vi "Vision Assistant.vi"(0 "Color Plane (Color Plane Extraction 1)":i32(ring)=2 items=["Red", "Green", "Blue", "Hue", "Saturation", "Luminance", "Value", "Intensity"], 1 "Range (Threshold 1)":cluster{"Lower value":sgl, "Upper value":sgl}={"Lower value"=199.0, "Upper value"=255.0}, 2 "Number of Erosion (Adv. Morphology 1)":i32=1, 3 "Square/Hexa (Square) (Adv. Morphology 1)":bool, 4 "Connectivity 4/8 (8) (Adv. Morphology 1)":bool=TRUE, 5 "Low Pass/High Pass (Low) (Adv. Morphology 1)":bool, 7 "error in":errorcluster) -> (20 "Number of Matches (Shape Matching 1)":i32, 21 "Shape Report (calibrated) (Shape Matching 1)":T2(array[cluster]) {"Score" format="%.2f"; "Centroid"."y" format="%.2f"; "Centroid"."x" format="%.2f"}, 27 "error out":errorcluster)   [LabVIEW 2016]
uses:
  <vilib>/vision/NI_Vision_Development_Module.lvlib
panel:
  out "Image Out":T1(plugin-control)
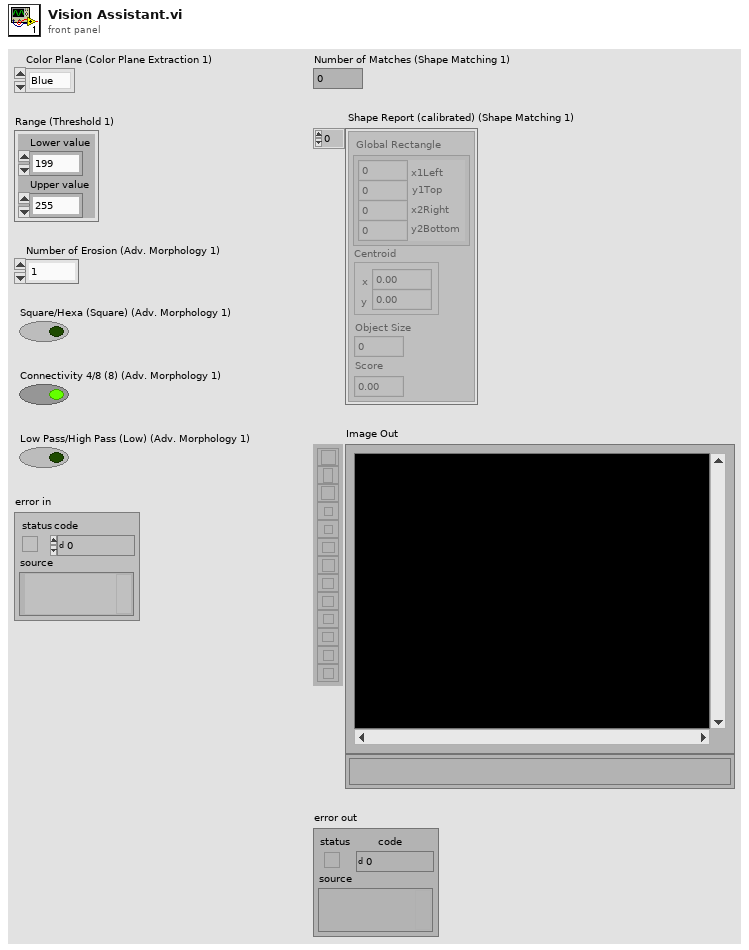
[diagram p1: front panel]
types:
  T1 = typedef "IMAQ Image.ctl" = refnum<image>
  T2 = cluster{"Global Rectangle":cluster{"x1Left":i32, "y1Top":i32, "x2Right":i32, "y2Bottom":i32}, "Centroid":cluster{"x":sgl, "y":sgl}, "Object Size":u32, "Score":dbl}[]
  T3 = typedef "Image Type" = u32
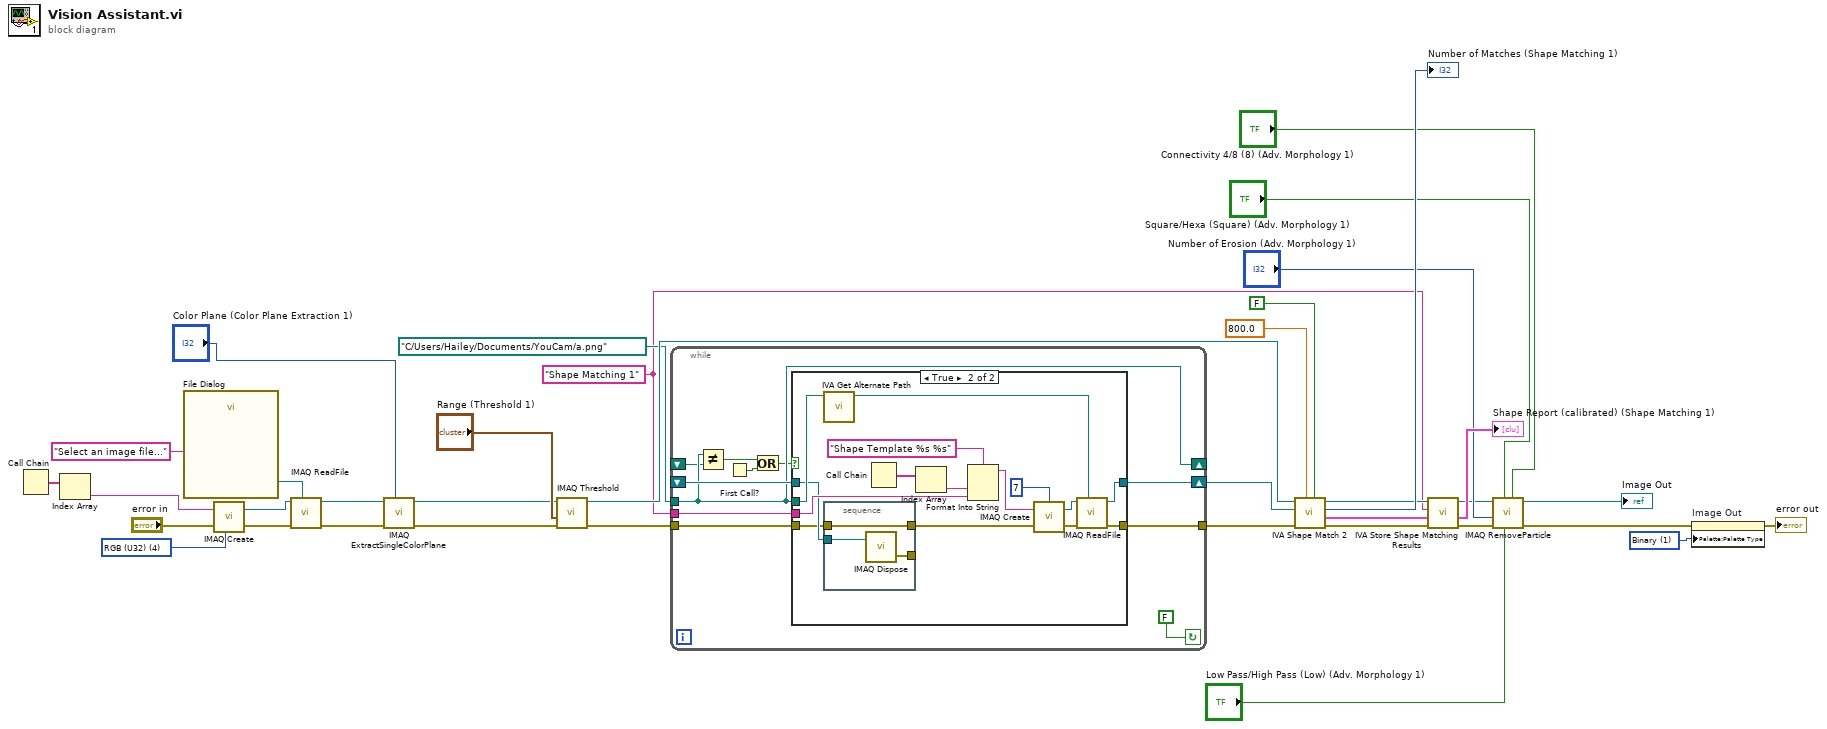
[diagram p0: block diagram]
diagram:
  w1 = u32 1 items=["Grayscale", "Binary", "Gradient", "Rainbow", "Temperature", "User Defined", "Binary 16 Bit", "Gradient 16 Bit", "Rainbow 16 Bit", "Temperature 16 Bit", "User Defined 16 Bit"] ("Palette Type")
  w10 = "Shape Matching 1" ("Step Name")
  w29 = T3 4 items=["Grayscale (U8)", "Grayscale (I16)", "Grayscale (SGL)", "Complex (CSG)", "RGB (U32)", "HSL (U32)", "RGB (U64)", "Grayscale (U16)"] ("Image Type")
  n1 = Call Chain() -> (call chain=w33:string[])
  n2 = Index Array(array=w33) -> (element=w32:string)  [unwired: 1 in]
  n3 = call "File Dialog"("prompt"="Select an image file...") -> ("selected path"=w30:path)  [unwired: 6 in, 8 out]
  n4 = call "IMAQ Create"("Image Name"=w32, "Image Type"=w29, "error in (no error)"="error in") -> ("New Image"=w36:T1, "error out"=w35:errorcluster)  [unwired: 1 in, 1 out]
  n5 = call "IMAQ ReadFile"("File Path"=w30, "error in (no error)"=w35, "Image"=w36) -> ("error out"=w37:errorcluster, "Image Out"=w27:T1)  [unwired: 2 in, 5 out]
  n6 = call "IMAQ ExtractSingleColorPlane"("Color Plane"="Color Plane (Color Plane Extraction 1)", "error in (no error)"=w37, "Image Src"=w27) -> ("error out"=w26:errorcluster, "Image Dst Out"=w24:T1)  [unwired: 1 in, 6 out]
  n7 = call "IMAQ Threshold"("error in (no error)"=w26, "Range"="Range (Threshold 1)", "Image Src"=w24) -> ("error out"=w23:errorcluster, "Image Dst Out"=w19:T1)  [unwired: 3 in, 4 out]
  n8 = while {
    shift-right: [w48] -> w11
    shift-left: _ -> [w47]
    tunnel: [w45] -> w12
    tunnel: w23 -> [w44]
    tunnel: path "C:/Users/Hailey/Documents/YouCam/a.png" ("Template Path") -> [w42]
    tunnel: w10 -> [w43]
    shift-right: [w42] -> _
    shift-left: _ -> [w41]
    stop <- FALSE continue-if-true
    n9 = Not Equal?(x=w42, y=w41) -> (x != y?=w39:bool)
    n10 = First Call?() -> (First Call?: T/F=w40:bool)
    n11 = Or(x=w39, y=w40) -> (x .or. y?=w38:bool)
    n12 = case shown="True" w38 {
      tunnel: [w50 w62] -> w48
      tunnel: w47 -> [w50 w53]
      tunnel: [w49 w60] -> w45
      tunnel: w44 -> [w49 w52]
      tunnel: w42 -> [_ w55]
      tunnel: w43 -> [_ w56]
      frame False {
      }
      frame True {
        n13 = call <vilib>:"IVA Get Alternate Path.vi"("Path In"=w55) -> ("Path Out"=w54:path)  [unwired: 10 out]
        n14 = stacked-sequence {
          tunnel: w53 -> [w68]
          tunnel: w52 -> [w67]
          tunnel: [w67] -> w51
          tunnel: [w66] -> _
          frame #0 {
            n15 = call "IMAQ Dispose"("Image"=w68) -> ("error out"=w66:errorcluster)  [unwired: 2 in, 3 out]
          }
        }
        n16 = Call Chain() -> (call chain=w58:string[])
        n17 = Index Array(array=w58) -> (element=w57:string)  [unwired: 1 in]
        n18 = Format Into String(format string="Shape Template %s %s" ("Image Name"), w57, w56) -> (resulting string=w65:string)  [unwired: 2 in, 1 out]
        n19 = call "IMAQ Create"("Border Size"=7, "Image Name"=w65, "error in (no error)"=w51) -> ("New Image"=w63:T1, "error out"=w61:errorcluster)  [unwired: 1 in, 1 out]
        n20 = call "IMAQ ReadFile"("File Path"=w54, "error in (no error)"=w61, "Image"=w63) -> ("error out"=w60:errorcluster, "Image Out"=w62:T1)  [unwired: 2 in, 5 out]
      }
    }
  }
  n21 = call <vilib>:"IVA Shape Match 2.vi"("Scale Invariance"=FALSE, "Minimal Score"=800.0, "error in (no error)"=w12, "Template"=w11, "Image Src"=w19) -> ("error out"=w18:errorcluster, "Shape Report"=w16:T2, "Number of Matches"=→"Number of Matches (Shape Matching 1)":i32, "Image Out"=w15:T1)  [unwired: 3 out]
  n22 = call <vilib>:"IVA Store Shape Matching Results.vi"("error in (no error)"=w18, "Shape Report"=w16, "Step Name"=w10, "Image in"=w15) -> ("error out"=w17:errorcluster, "Shape Report (calibrated)"=→"Shape Report (calibrated) (Shape Matching 1)":T2, "Image dup"=w5:T1)  [unwired: 5 out]
  n23 = call "IMAQ RemoveParticle"("Connectivity 4/8 (8)"="Connectivity 4/8 (8) (Adv. Morphology 1)", "Low Pass/High Pass (Low)"="Low Pass/High Pass (Low) (Adv. Morphology 1)", "Square/Hexa (Square)"="Square/Hexa (Square) (Adv. Morphology 1)", "error in (no error)"=w17, "Number of Erosion"="Number of Erosion (Adv. Morphology 1)", "Image Src"=w5) -> ("error out"=w4:errorcluster, "Image Dst Out"=→"Image Out":T1)  [unwired: 1 in, 3 out]
  n24 = property on="Image Out" class="ImageControl"(error in=w4, "Palette:Palette Type"=w1) -> (error out=→"error out":errorcluster)  [unwired: 1 in, 1 out]
